vi "Find Ballard MIL-STD-1553 Custom Device.vi"(8 "error in":errorcluster, 10 "name":string, 11 "target in":refnum<k24>) -> (0 "error out":errorcluster, 2 "Ballard MIL-STD 1553 custom device":T1 format="%.0x", 3 "target out":refnum<k24>, 4 "found?":bool)   [LabVIEW 2020, in "AIM MIL-STD-1553 Scripting.lvlib"]
doc: "Within the specified target, this VI searches for the named Ballard MIL-STD-1553 custom device and returns a reference to the found <b>Ballard MIL-STD-1553 custom device</b>."
uses:
  AIM MIL-STD-1553 Scripting.lvlib
  NationalInstruments.VeriStand.SystemDefinitionAPI
  Constants.vi
  <vilib>/NI VeriStand/Custom Device API/Custom Device Item Ref.ctl
  <vilib>/NI VeriStand/Custom Device API/Custom Device API.lvlib
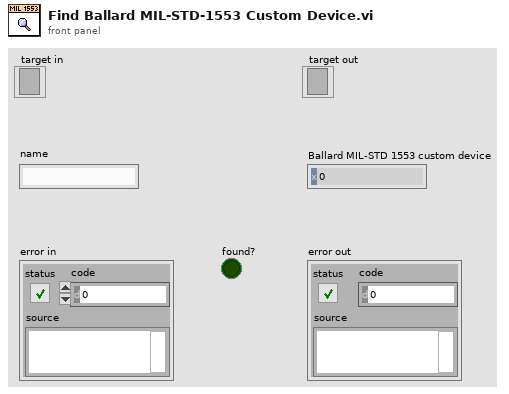
[diagram p1: front panel]
types:
  T1 = typedef "Custom Device API.lvlib/Custom Device Item Ref.ctl" = u64
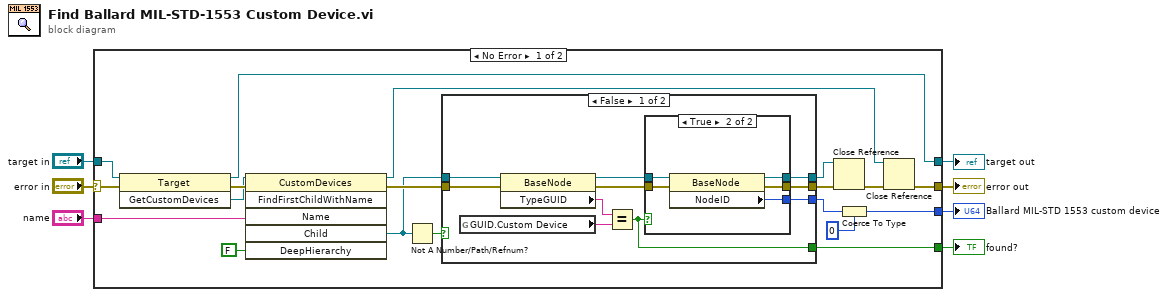
[diagram p0: block diagram]
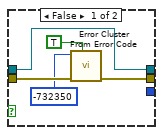
[diagram p2: hidden frame]
diagram:
  n1 = case shown="No Error" "error in" {
    selector: "error in" -> [w21 w50]
    tunnel: "target in" -> [w22 w49]
    tunnel: [w16 w50] -> w5
    tunnel: [w9 _] -> w2
    tunnel: [w18 w49] -> w4
    tunnel: "name" -> [w15 _]
    tunnel: [w11 _] -> w1
    frame No Error {
      n2 = invoke on="Invoke Node" class="Target" method="GetCustomDevices"(reference=w22, error in=w21) -> (reference out=w18:refnum<k24>, error out=w26:errorcluster, "GetCustomDevices"=w25:refnum<k24>)  [unwired: 1 in]
      n3 = invoke on="Invoke Node" class="CustomDevices" method="FindFirstChildWithName"(reference=w25, error in=w26, "Name"=w15, "DeepHierarchy"=FALSE) -> (reference out=w19:refnum<k24>, error out=w17:errorcluster, "Child"=w14:refnum<k24>)  [unwired: 2 in, 3 out]
      n4 = Not A Number/Path/Refnum?(number/path/refnum=w14) -> (NaN/Path/Refnum?=w13:bool)
      n5 = case shown="False" w13 {
        tunnel: [w36 w47] -> w24
        tunnel: [w35 w48] -> w23
        tunnel: w17 -> [w33 w48]
        tunnel: w14 -> [w32 w47]
        tunnel: [w34 _] -> w10
        tunnel: [w27 _] -> w11
        frame False {
          n6 = global read "Constants.vi" "GUID.Custom Device"() -> (w30:string)
          n7 = property on="Property Node" class="BaseNode"(reference=w32, error in=w33) -> (reference out=w28:refnum<k24>, error out=w29:errorcluster, "TypeGUID"=w31:string)
          n8 = Equal?(x=w31, y=w30) -> (x = y?=w27:bool)
          n9 = case shown="True" w27 {
            tunnel: [w38 w43] -> w35
            tunnel: w29 -> [w40 w45]
            tunnel: w28 -> [w41 w46]
            tunnel: [w41 w44] -> w36
            tunnel: [_ w42] -> w34
            frame False {
              n10 = call <vilib>:"Error Cluster From Error Code.vi"("show call chain? (False)"=TRUE, "error in (no error)"=w40, "error code (0)"=-732350) -> ("error out"=w38:errorcluster)  [unwired: 6 in]
            }
            frame True {
              n11 = property on="Property Node" class="BaseNode"(reference=w46, error in=w45) -> (reference out=w44:refnum<k24>, error out=w43:errorcluster, "NodeID"=w42:u64)
            }
          }
        }
        frame True {
        }
      }
      n12 = Close Reference(reference=w24, error in (no error)=w23) -> (error out=w20:errorcluster)
      n13 = Coerce To Type(0:w10, 1:T1 0 ("Ballard MIL-STD 1553 custom device")) -> (2:w9:T1)
      n14 = Close Reference(reference=w19, error in (no error)=w20) -> (error out=w16:errorcluster)
    }
    frame Error {
    }
  }
  "error out" <- w5
  "target out" <- w4
  "Ballard MIL-STD 1553 custom device" <- w2
  "found?" <- w1
